vi "sr-latch loop test.vi"() -> ()   [LabVIEW 2017]
panel:
  in  "Start":bool
  in  "pulse":bool
  out "2bit":bool
  out "3bit":bool
  out "1bit":bool
  out "0bit":bool
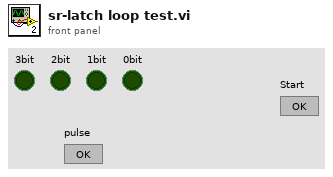
[diagram p1: front panel]
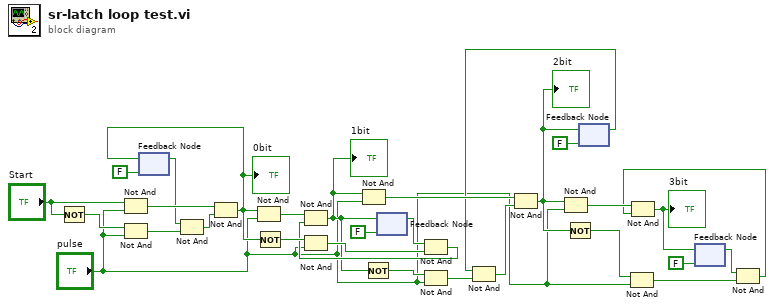
[diagram p0: block diagram]
diagram:
  n1 = Not(x="Start") -> (.not. x?=w30:bool)
  n2 = Not And(1:"pulse", 2:"Start") -> (0:w29:bool)
  n3 = Not And(1:"pulse", 2:w30) -> (0:w28:bool)
  n4 = feedback #1(FALSE) -> (w20:bool)
  n5 = Not And(1:w28, 2:w20) -> (0:w27:bool)
  n6 = Not And(1:w27, 2:w29) -> (0:w21:bool)
  "0bit" <- w21
  n7 = feedback-in #1(w21) -> ()
  n8 = Not And(1:"pulse", 2:w21) -> (0:w24:bool)
  n9 = Not(x=w21) -> (.not. x?=w25:bool)
  n10 = Not And(1:"pulse", 2:w25) -> (0:w23:bool)
  n11 = feedback #2(FALSE) -> (w18:bool)
  n12 = Not And(1:w23, 2:w18) -> (0:w22:bool)
  n13 = Not And(1:w22, 2:w24) -> (0:w10:bool)
  "1bit" <- w10
  n14 = Not And(1:"pulse", 2:w10) -> (0:w15:bool)
  n15 = Not(x=w10) -> (.not. x?=w16:bool)
  n16 = feedback-in #2(w10) -> ()
  n17 = Not And(1:"pulse", 2:w16) -> (0:w14:bool)
  n18 = feedback #3(FALSE) -> (w12:bool)
  n19 = Not And(1:w14, 2:w12) -> (0:w13:bool)
  n20 = Not And(1:w13, 2:w15) -> (0:w2:bool)
  "2bit" <- w2
  n21 = Not And(1:"pulse", 2:w2) -> (0:w8:bool)
  n22 = Not(x=w2) -> (.not. x?=w9:bool)
  n23 = feedback-in #3(w2) -> ()
  n24 = Not And(1:"pulse", 2:w9) -> (0:w7:bool)
  n25 = feedback #4(FALSE) -> (w5:bool)
  n26 = Not And(1:w7, 2:w5) -> (0:w6:bool)
  n27 = Not And(1:w6, 2:w8) -> (0:w3:bool)
  "3bit" <- w3
  n28 = feedback-in #4(w3) -> ()
